vi "VALEW_ATC_Verify Concurrent All Valves.vi"(0 "GEA2 Reference In":refnum<k24>, 11 "Error In":errorcluster) -> (4 "GEA2 Reference Out":refnum<k24>, 6 "Pass/fail?":bool, 8 "Report Text":string, 15 "Error Out":errorcluster)   [LabVIEW 2016, in "Centauro.lvlib"]
doc: "This test covers the ATC algorithm when doing a concurrent fill with ALL valves. A concurrent fill allows both hot and cold valves to be on at the same time. The valves are operated in parallel. When the cold valve is requested to be on, the fabric softener and spray valves also come on in this test."
uses:
  Projects/Centauro.lvlib
  Q:/Common/DLLs/GEA3/GeaCommunication.dll
  Common/DLLs/GEA3/GeaCommunication.dll
  Common/LabVIEW GEA2 Toolkit/LabVIEW_GEA2_Toolkit.lvlibp/type defs/Source_Destination.ctl
  Common/LabVIEW GEA2 Toolkit/LabVIEW_GEA2_Toolkit.lvlibp/type defs/ERD Write Data In.ctl
  Common/LabVIEW GEA2 Toolkit/LabVIEW_GEA2_Toolkit.lvlibp/type defs/Data Type.ctl
  Common/LabVIEW GEA2 Toolkit/LabVIEW_GEA2_Toolkit.lvlibp/type defs/ERD Read Data In.ctl
  Valew Common/type defs/MC_Cycle_Engine_Request_State.ctl
  <vilib>/DAQmx/write.llb/DAQmx Write (Analog DBL 1Chan 1Samp).vi
  <vilib>/DAQmx/create/channels.llb/DAQmx Create Channel (AO-Voltage-Basic).vi
  <vilib>/DAQmx/miscellaneous.llb/DAQmx Fill In Error Info.vi
  Common/LabVIEW GEA2 Toolkit/LabVIEW_GEA2_Toolkit.lvlibp
panel:
  out "Calc bath temp after seg gals":dbl
  out "Bath temp after seg gals":dbl
  out "Hot valve time (s) ATC":u16
  out "Cold valve time (s) ATC":u16
  out "Bath temp updated after segment fill?":bool
  out "Valve ON Times (s)":dbl[](array[numeric])
  out "Cold valve pass?":bool
  out "Hot valve pass?":bool
  out "Cold valve time (s) Calc":dbl
  out "Hot valve time (s) Calc":dbl
  in  "Standalone?":bool
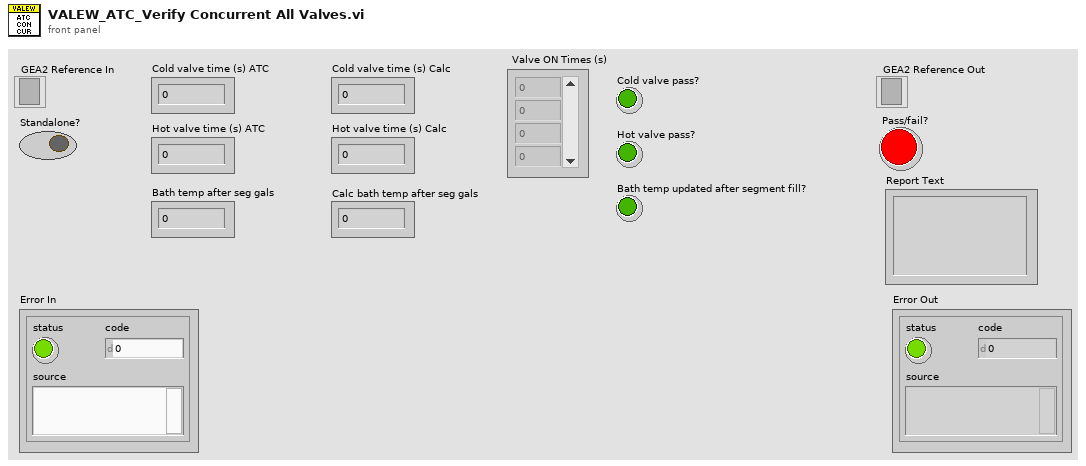
[diagram p1: front panel]
types:
  T1 = typedef "Centauro.lvlib/MC_Cycle_Engine_Request_State.ctl" = enum16{"Select", "Start", "Pause", "Resume", "Stop"}
  T2 = typedef "LabVIEW_GEA2_Toolkit.lvlibp/ERD Write Data In.ctl" = cluster{"ERD Number":u16, "Data Type":T3, "Data":string}
  T3 = typedef "LabVIEW_GEA2_Toolkit.lvlibp/Data Type.ctl" = enum16{"string", "boolean", "uint8_t", "uint16_t", "uint32_t", "uint64_t", "int8_t", "int16_t", "int32_t", "int64_t"}
  T4 = typedef "LabVIEW_GEA2_Toolkit.lvlibp/ERD Read Data In.ctl" = cluster{"ERD Number":u16, "Data Type":T3}
  T5 = enum16{"EQ (==)", "NE (!=)", "GT (>)", "LT (<)", "GE (>=)", "LE (<=)", "GTLT(> <)", "GELE (>= <=)", "GELT (>= <)", "GTLE (> <=)", "LTGT (< >)", "LEGE (<= >=)", "LEGT (<= >)", "LTGE (< >=)", "No Comparison"}
  T6 = typedef "LabVIEW_GEA2_Toolkit.lvlibp/Source_Destination.ctl" = cluster{"Source":u8, "Destination":u8}
  T7 = typedef "Centauro.lvlib/VALEW_ATC_Data.ctl" = cluster{"Accumulated hot gallons":dbl, "Accumulated cold gallons":dbl, "Current tub gallons":dbl, "Cold inlet temp (F)":dbl, "Hot inlet temp (F)":dbl, "Warm inlet temp (F)":dbl, "Hot valve time (s)":u16, "Cold valve time (s)":u16, "Current bath temp (F)":dbl, "Current water temp (F)":dbl, "Segment gallons":dbl}
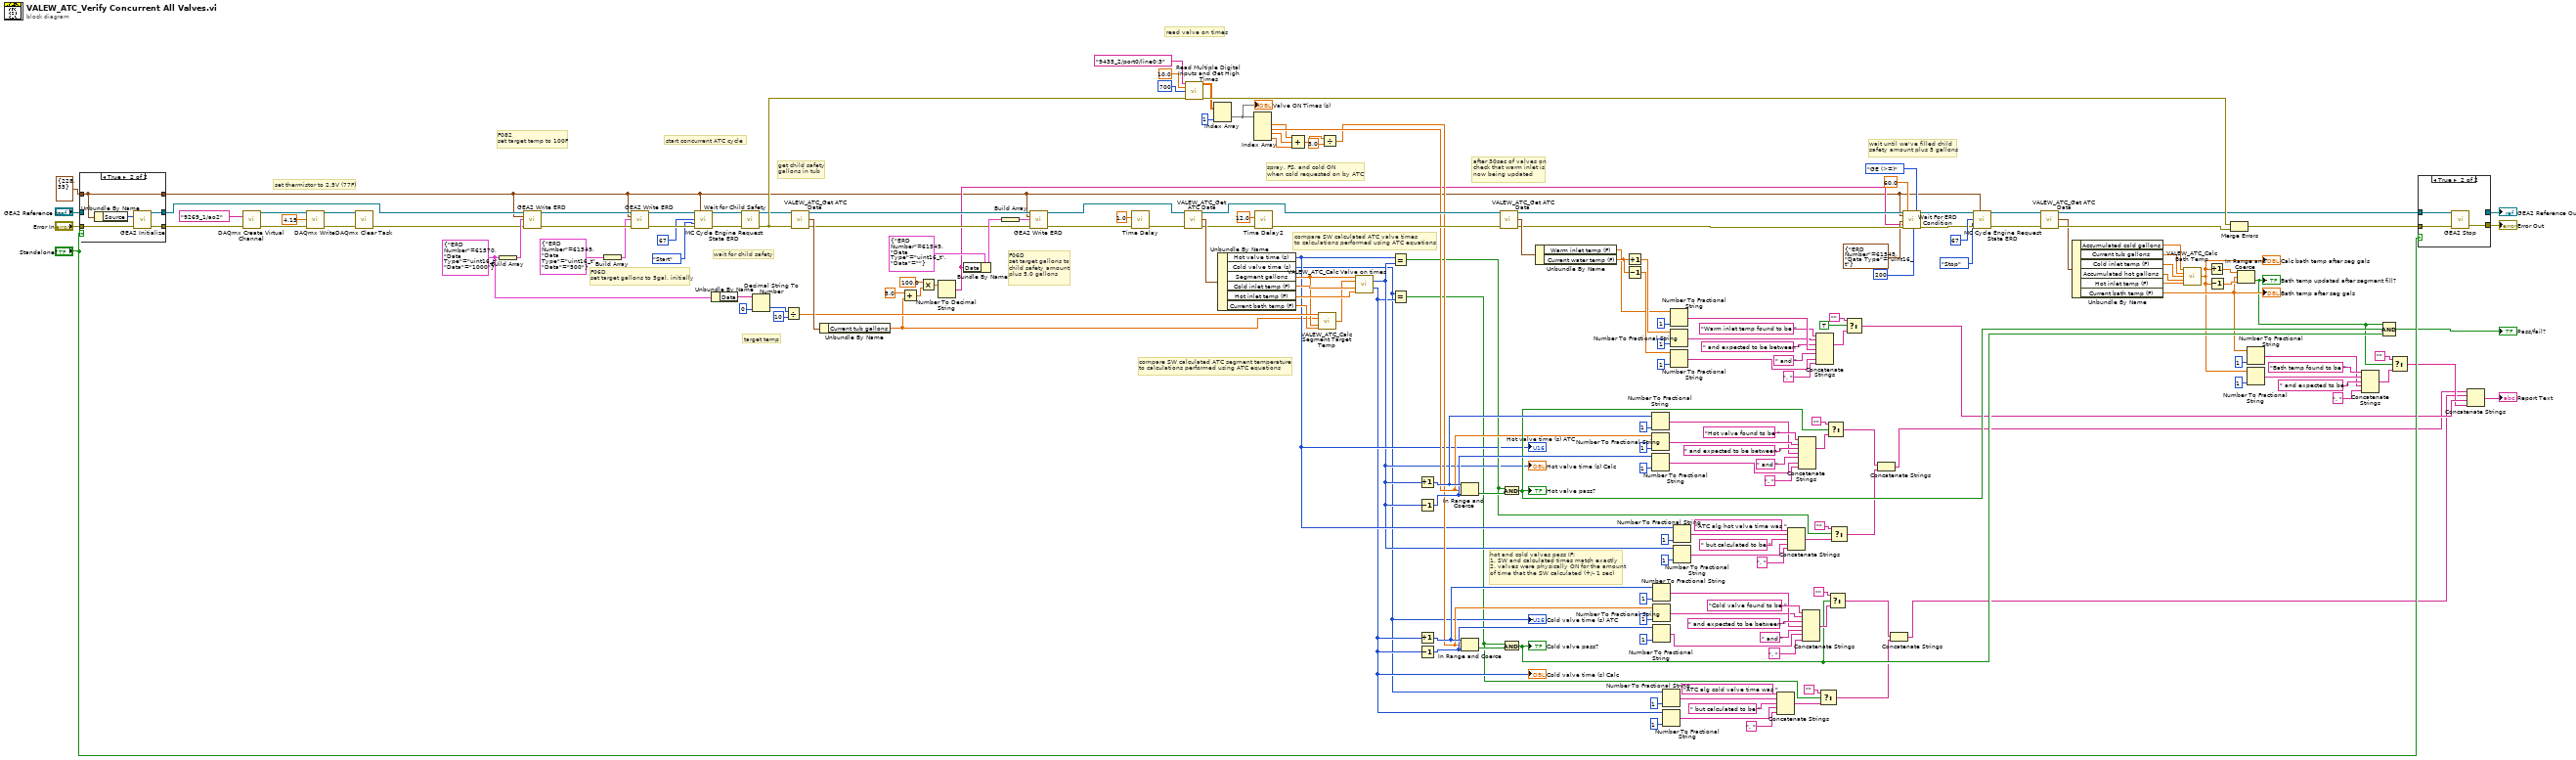
[diagram p0: block diagram]
diagram:
  w187 = T2 {"ERD Number"=61570, "Data Type"=enum."uint16_t", "Data"="1000"} ("ERD Write Data In")
  # "hot and cold valves pass IF:\n1. SW and calculated times match exactly\n2. valves were physically ON for the amount\nof time that the SW calculated (+/- 1 sec)"
  # "compare SW calculated ATC segment temperature\nto calculations performed using ATC equations"
  # "compare SW calculated ATC valve times\nto calculations performed using ATC equations"
  # "F06D\nset target gallons to\nchild safety amount\nplus 5.0 gallons"
  # "spray, FS, and cold ON\nwhen cold requested on by ATC"
  # "F06D\nset target gallons to 5gal, initially"
  # "after 30sec of valves on\ncheck that warm inlet is\nnow being updated"
  # "get child safety\ngallons in tub"
  # "wait until we've filled child \nsafety amount plus 5 gallons"
  # "read valve on times"
  # "target temp"
  # "set thermistor to 2.5V (77F)"
  # "wait for child safety"
  # "start concurrent ATC cycle"
  # "F082\nset target temp to 100F"
  n1 = case shown="True" "Standalone?" {
    tunnel: T6 {"Source"=228, "Destination"=35} ("GEA Inputs") -> [w195 w198]
    tunnel: [w197 w201] -> w56
    tunnel: [w196 w200] -> w145
    tunnel: "Error In" -> [w196 w199]
    tunnel: "GEA2 Reference In" -> [w197 _]
    tunnel: [w195 w198] -> w5
    frame False {
    }
    frame True {
      n2 = Unbundle By Name(w198) -> ("Source"=w202:u8)
      n3 = call "GEA2 Initialize.vi"("Source Address"=w202, "error in"=w199) -> ("GEA2 Reference Out"=w201:refnum<k24>, "error out"=w200:errorcluster)  [unwired: 11 in, 1 out]
    }
  }
  n4 = call-poly <vilib>:"DAQmx Create Virtual Channel.vi"("physical channels"=tag "9269_1/ao2", "error in"=w145) -> ("task out"=w173:refnum<k21>, "error out"=w172:errorcluster)  [unwired: 12 in]
  n5 = call-poly <vilib>:"DAQmx Write.vi"("task/channels in"=w173, "data"=4.15, "error in"=w172) -> ("task out"=w143:refnum<k21>, "error out"=w144:errorcluster)  [unwired: 10 in, 1 out]
  n6 = call <vilib>:"DAQmx Clear Task.vi"("task in"=w143, "error in"=w144) -> ("error out"=w57:errorcluster)  [unwired: 13 in]
  n7 = Build Array(w187) -> (w186:T2[])
  n8 = call "GEA2 Write ERD.vi"("GEA2 Reference In"=w56, "GEA Inputs"=w5, "Write ERD List"=w186, "Error In"=w57) -> ("GEA2 Reference Out"=w168:refnum<k24>, "Error Out"=w167:errorcluster)  [unwired: 9 in, 1 out]
  n9 = Build Array(T2 {"ERD Number"=61549, "Data Type"=enum."uint16_t", "Data"="500"} ("ERD Write Data In")) -> (w138:T2[])
  n10 = call "GEA2 Write ERD.vi"("GEA2 Reference In"=w168, "GEA Inputs"=w5, "Write ERD List"=w138, "Error In"=w167) -> ("GEA2 Reference Out"=w6:refnum<k24>, "Error Out"=w7:errorcluster)  [unwired: 9 in, 1 out]
  n11 = call "MC Cycle Engine Request State ERD.vi"("GEA2 Reference In"=w6, "GEA Inputs"=w5, "Cycle #"=u8 67, "MC Cycle Engine State"=MC_Cycle_Engine_Request_State."Start", "Error In"=w7) -> ("GEA2 Reference Out"=w10:refnum<k24>, "Error Out"=w8:errorcluster)  [unwired: 9 in]
  n12 = Unbundle By Name(w187) -> ("Data"=w185:string)
  n13 = call "Wait for Child Safety.vi"("GEA2 Reference In"=w10, "Error In"=w8) -> ("GEA2 Reference Out"=w2:refnum<k24>, "Error Out"=w9:errorcluster)  [unwired: 9 in, 3 out]
  n14 = Decimal String To Number(string=w185, default (0L)=u16 0 ("default (0 U32)")) -> (number=w183:u16)  [unwired: 1 in, 1 out]
  n15 = Divide(x=w183, y=u16 10) -> (x/y=w141:dbl)
  n16 = call "VALEW_ATC_Get ATC Data.vi"("GEA2 Reference In"=w2, "Error In"=w9) -> ("GEA2 Reference Out"=w18:refnum<k24>, "ATC Data"=w166:T7, "Error Out"=w17:errorcluster)  [unwired: 11 in]
  n17 = Unbundle By Name(w166) -> ("Current tub gallons"=w14:dbl)
  n18 = Add(x=5.0, y=w14) -> (x+y=w20:dbl)
  n19 = Multiply(x=100.0, y=w20) -> (x*y=w21:dbl)
  n20 = Number To Decimal String(number=w21) -> (decimal integer string=w13:string)  [unwired: 1 in]
  n21 = Bundle By Name(cluster=T2 {"ERD Number"=61549, "Data Type"=enum."uint16_t", "Data"=""} ("ERD Write Data In"), "Data"=w13) -> (w22:T2)
  n22 = Build Array(w22) -> (w25:T2[])
  n23 = call "GEA2 Write ERD.vi"("GEA2 Reference In"=w18, "GEA Inputs"=w5, "Write ERD List"=w25, "Error In"=w17) -> ("GEA2 Reference Out"=w16:refnum<k24>, "Error Out"=w15:errorcluster)  [unwired: 9 in, 1 out]
  n24 = call "Time Delay"("error in (no error)"=w15, "Delay Time (s)"=1.0) -> ("error out"=w190:errorcluster)  [unwired: 9 in]
  n25 = call "VALEW_ATC_Get ATC Data.vi"("GEA2 Reference In"=w16, "Error In"=w190) -> ("GEA2 Reference Out"=w175:refnum<k24>, "ATC Data"=w189:T7, "Error Out"=w177:errorcluster)  [unwired: 11 in]
  n26 = call "Read Multiple Digital Inputs and Get High Times.vi"("Lines"=tag "9435_2/port0/line0:3", "Rate (Hz)"=10.0 ("rate"), "Samples"=700 ("samples per channel"), "Error In"=w9) -> ("High Times (s)"=w156:dbl[][], "Error Out"=w169:errorcluster)  [unwired: 10 in]
  n27 = Index Array(array=w156, index (col)=1 ("disabled index (col)")) -> (element=w71:dbl[])  [unwired: 1 in]
  "Valve ON Times (s)" <- w71
  n28 = Unbundle By Name(w189) -> ("Hot valve time (s)"=w42:u16, "Cold valve time (s)"=w30:u16, "Segment gallons"=w140:dbl, "Cold inlet temp (F)"=w157:dbl, "Hot inlet temp (F)"=w188:dbl, "Current bath temp (F)"=w139:dbl)
  "Cold valve time (s) ATC" <- w30
  "Hot valve time (s) ATC" <- w42
  n29 = Index Array(array=w71) -> (element #1=w65:dbl, element #2=w70:dbl, element #3=w69:dbl, element #4=w68:dbl)  [unwired: 4 in]
  n30 = call "Time Delay2"("error in (no error)"=w177, "Delay Time (s)"=12.0) -> ("error out"=w176:errorcluster)  [unwired: 9 in]
  n31 = Compound Arithmetic op=ADD(w65, w69, w68) -> (w67:dbl)
  n32 = call "VALEW_ATC_Calc Segment Target Temp.vi"("T(target)"=w141, "V(bath)"=w14, "V(segment)"=w140, "T(bath)"=w139) -> ("T(segment target)"=w142:dbl)  [unwired: 11 in]
  n33 = Divide(x=w67, y=3.0) -> (x/y=w64:dbl)
  n34 = call "VALEW_ATC_Calc Valve on times.vi"("V(segment)"=w140, "T(segment target)"=w142, "T(cold inlet)"=w157, "T(hot inlet)"=w188) -> ("t(hot valve)"=w41:u16, "t(cold valve)"=w31:u16)  [unwired: 10 in]
  "Hot valve time (s) Calc" <- w41
  "Cold valve time (s) Calc" <- w31
  n35 = Equal?(x=w42, y=w41) -> (x = y?=w43:bool)
  n36 = Equal?(x=w30, y=w31) -> (x = y?=w29:bool)
  n37 = Increment(x=w41) -> (x+1=w132:u16)
  n38 = Decrement(x=w41) -> (x-1=w127:u16)
  n39 = Increment(x=w31) -> (x+1=w125:u16)
  n40 = Decrement(x=w31) -> (x-1=w124:u16)
  n41 = In Range and Coerce(upper limit=w132, x=w70, lower limit=w127) -> (In Range?=w155:bool)  [unwired: 1 out]
  n42 = In Range and Coerce(upper limit=w125, x=w64, lower limit=w124) -> (In Range?=w154:bool)  [unwired: 1 out]
  n43 = call "VALEW_ATC_Get ATC Data.vi"("GEA2 Reference In"=w175, "Error In"=w176) -> ("GEA2 Reference Out"=w164:refnum<k24>, "ATC Data"=w174:T7, "Error Out"=w165:errorcluster)  [unwired: 11 in]
  n44 = And(x=w43, y=w155) -> (x .and. y?=w107:bool)
  "Hot valve pass?" <- w107
  n45 = And(x=w29, y=w154) -> (x .and. y?=w106:bool)
  "Cold valve pass?" <- w106
  n46 = Unbundle By Name(w174) -> ("Warm inlet temp (F)"=w12:dbl, "Current water temp (F)"=w153:dbl)
  n47 = Increment(x=w153) -> (x+1=w92:dbl)
  n48 = Decrement(x=w153) -> (x-1=w91:dbl)
  n49 = Number To Fractional String(number=w132, precision (6)=i16 1) -> (F-format string=w120:string)  [unwired: 2 in]
  n50 = Number To Fractional String(number=w70, precision (6)=i16 1) -> (F-format string=w122:string)  [unwired: 2 in]
  n51 = Number To Fractional String(number=w127, precision (6)=i16 1) -> (F-format string=w118:string)  [unwired: 2 in]
  n52 = Number To Fractional String(number=w125, precision (6)=i16 1) -> (F-format string=w111:string)  [unwired: 2 in]
  n53 = Number To Fractional String(number=w64, precision (6)=i16 1) -> (F-format string=w110:string)  [unwired: 2 in]
  n54 = Number To Fractional String(number=w124, precision (6)=i16 1) -> (F-format string=w109:string)  [unwired: 2 in]
  n55 = Number To Fractional String(number=w30, precision (6)=i16 1) -> (F-format string=w35:string)  [unwired: 2 in]
  n56 = Number To Fractional String(number=w31, precision (6)=i16 1) -> (F-format string=w37:string)  [unwired: 2 in]
  n57 = Number To Fractional String(number=w12, precision (6)=i16 1) -> (F-format string=w100:string)  [unwired: 2 in]
  n58 = Number To Fractional String(number=w92, precision (6)=i16 1) -> (F-format string=w98:string)  [unwired: 2 in]
  n59 = Number To Fractional String(number=w91, precision (6)=i16 1) -> (F-format string=w102:string)  [unwired: 2 in]
  n60 = Number To Fractional String(number=w42, precision (6)=i16 1) -> (F-format string=w53:string)  [unwired: 2 in]
  n61 = Number To Fractional String(number=w41, precision (6)=i16 1) -> (F-format string=w51:string)  [unwired: 2 in]
  n62 = Concatenate Strings("ATC alg cold valve time was ", w35, " but calculated to be ", w37, ". " ("string")) -> (w40:string)
  n63 = Concatenate Strings("ATC alg hot valve time was ", w53, " but calculated to be ", w51, ". " ("string")) -> (w48:string)
  n64 = Concatenate Strings("Hot valve found to be ", w122, " and expected to be between ", w120, " and " ("string"), w118, ". " ("string")) -> (w116:string)
  n65 = Concatenate Strings("Cold valve found to be ", w110, " and expected to be between ", w111, " and " ("string"), w109, ". " ("string")) -> (w108:string)
  n66 = Concatenate Strings("Warm inlet temp found to be ", w98, " and expected to be between ", w100, " and " ("string"), w102, ". " ("string")) -> (w104:string)
  n67 = Select(t="", s=w29, f=w40) -> (s? t:f=w28:string)
  n68 = Select(t="", s=w107, f=w116) -> (s? t:f=w45:string)
  n69 = Select(t="", s=w106, f=w108) -> (s? t:f=w27:string)
  n70 = Select(t="", s=w43, f=w48) -> (s? t:f=w46:string)
  n71 = Select(t="", s=TRUE, f=w104) -> (s? t:f=w78:string)
  n72 = Concatenate Strings(w45, w46) -> (w44:string)
  n73 = Concatenate Strings(w27, w28) -> (w26:string)
  n74 = call "Wait For ERD Condition.vi"("GEA2 Reference In"=w164, "GEA Inputs"=w5, "ERD Read Data"=T4 {"ERD Number"=61545, "Data Type"=enum."uint16_t"}, "Expected Low"=w13, "Error In"=w165, "Timeout (s)"=60.0, "Loop Rate (ms)"=u32 200, "Comparison"=T5."GE (>=)") -> ("GEA2 Reference Out"=w63:refnum<k24>, "Error Out"=w60:errorcluster)  [unwired: 7 in, 3 out]
  n75 = call "MC Cycle Engine Request State ERD.vi"("GEA2 Reference In"=w63, "GEA Inputs"=w5, "Cycle #"=u8 67, "MC Cycle Engine State"=MC_Cycle_Engine_Request_State."Stop", "Error In"=w60) -> ("GEA2 Reference Out"=w62:refnum<k24>, "Error Out"=w61:errorcluster)  [unwired: 9 in]
  n76 = call "VALEW_ATC_Get ATC Data.vi"("GEA2 Reference In"=w62, "Error In"=w61) -> ("GEA2 Reference Out"=w59:refnum<k24>, "ATC Data"=w158:T7, "Error Out"=w159:errorcluster)  [unwired: 11 in]
  n77 = Unbundle By Name(w158) -> ("Accumulated cold gallons"=w148:dbl, "Current tub gallons"=w149:dbl, "Cold inlet temp (F)"=w150:dbl, "Accumulated hot gallons"=w151:dbl, "Hot inlet temp (F)"=w152:dbl, "Current bath temp (F)"=w82:dbl)
  "Bath temp after seg gals" <- w82
  n78 = call "VALEW_ATC_Calc Bath Temp.vi"("V(bath cold)"=w148, "V(bath)"=w149, "T(cold inlet)"=w150, "V(bath hot)"=w151, "T(hot inlet)"=w152) -> ("T(bath)"=w81:dbl)  [unwired: 10 in]
  "Calc bath temp after seg gals" <- w81
  n79 = Increment(x=w81) -> (x+1=w146:dbl)
  n80 = Decrement(x=w81) -> (x-1=w147:dbl)
  n81 = Merge Errors(w169, w159) -> (w58:errorcluster)
  n82 = In Range and Coerce(upper limit=w146, x=w82, lower limit=w147) -> (In Range?=w79:bool)  [unwired: 1 out]
  "Bath temp updated after segment fill?" <- w79
  n83 = Number To Fractional String(number=w82, precision (6)=i16 1) -> (F-format string=w84:string)  [unwired: 2 in]
  n84 = Number To Fractional String(number=w81, precision (6)=i16 1) -> (F-format string=w86:string)  [unwired: 2 in]
  n85 = Concatenate Strings("Bath temp found to be ", w86, " and expected to be ", w84, ". " ("string")) -> (w83:string)
  n86 = Compound Arithmetic op=AND(w79, w107, w106) -> (→"Pass/fail?":bool)
  n87 = Select(t="", s=w79, f=w83) -> (s? t:f=w77:string)
  n88 = case shown="True" "Standalone?" {
    tunnel: w58 -> [w204 w207]
    tunnel: w59 -> [w203 w206]
    tunnel: [w204 w205] -> w75
    tunnel: [w203 _] -> w136
    frame False {
    }
    frame True {
      n89 = call "GEA2 Stop.vi"("GEA2 Reference In"=w206, "Error In"=w207) -> ("Error Out"=w205:errorcluster)  [unwired: 13 in]
    }
  }
  "GEA2 Reference Out" <- w136
  "Error Out" <- w75
  n90 = Concatenate Strings(w44, w26, w78, w77) -> (→"Report Text":string)
